vi "Generate Register 0 Write Vectors.vi"(0 "Slave Address":T2=12 format="%02x", 1 "Alias":string, 5 "Register Data":T1 format="%02x", 11 "error in (no error)":errorcluster) -> (4 "Vector Statements":string[](array[string]), 15 "error out":errorcluster)   [LabVIEW 2018, in "MIPI RFFE API.lvlib"]
uses:
  MIPI RFFE API.lvlib
  Slave Address.ctl
  Register Data.ctl
  Reg0Write/RFFE Reg0Write Command.lvclass
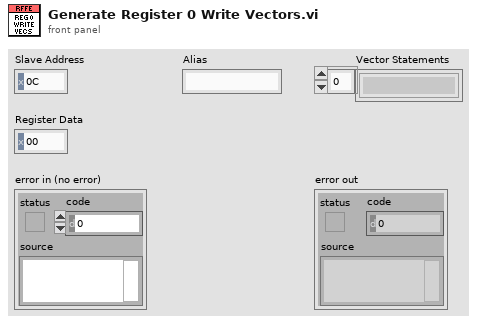
[diagram p1: front panel]
types:
  T1 = typedef "MIPI RFFE API.lvlib/Register Data.ctl" = u8
  T2 = typedef "MIPI RFFE API.lvlib/Slave Address.ctl" = u8
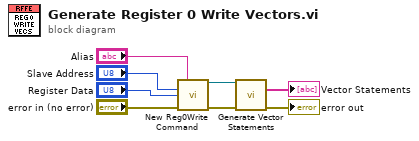
[diagram p0: block diagram]
diagram:
  n1 = call "New Reg0Write Command.vi"("Alias"="Alias", "Slave Address"="Slave Address", "Register Data"="Register Data", "error in (no error)"="error in (no error)") -> ("RFFE Reg0Write Command out"=w3:refnum<class "RFFE Reg0Write Command.lvclass">, "error out"=w2:errorcluster)  [unwired: 10 in]
  n2 = call-dynamic "Generate Vector Statements.vi"("RFFE Command in"=w3, "error in (no error)"=w2) -> ("Vector Statements"=→"Vector Statements":string[], "error out"=→"error out":errorcluster)  [unwired: 11 in, 1 out]
